vi "Load Microphone 2D Locations.vi"(3 "error in":errorcluster, 4 "Sensor Locations File":path=path "C:/Users/plane/Desktop/MTA/SCM with Cu Windows.cfg") -> (0 "error out":errorcluster, 1 "data":cluster{"r":dbl, "theta":dbl}[](array[cluster]))   [LabVIEW 2013]
panel:
  in  "Transducer Coordinates (cm, rad)":cluster{"r":dbl, "theta":dbl}[](array[cluster])
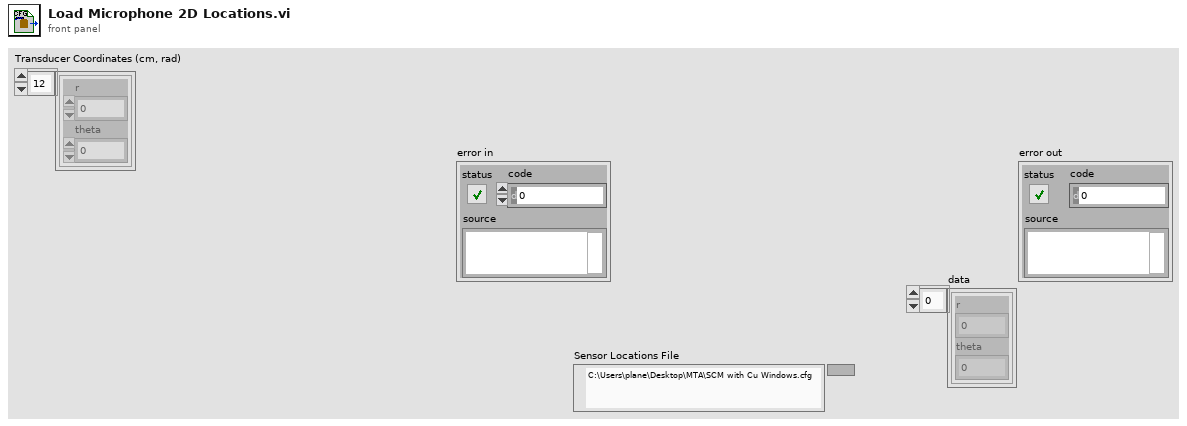
[diagram p1: front panel]
types:
  T1 = enum16{"big-endian, network order", "native, host order", "little-endian"}
  T2 = enum16{"open", "replace", "create", "open or create", "replace or create", "replace or create with confirmation"}
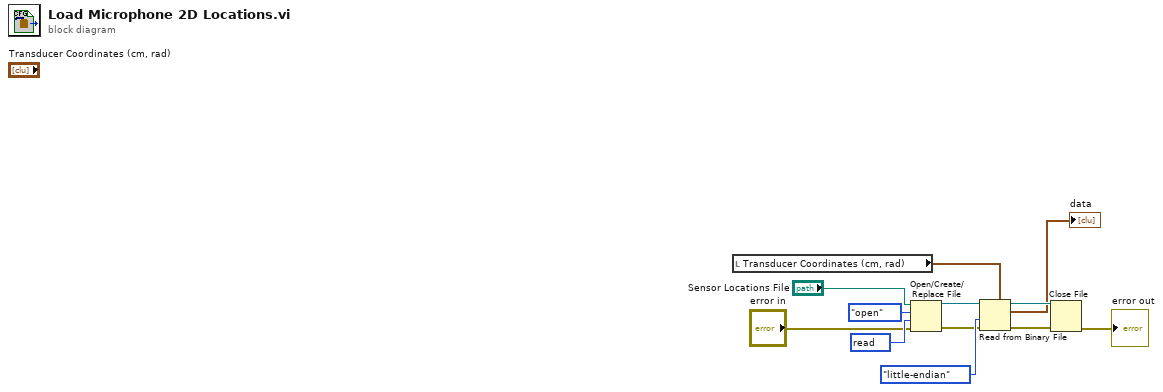
[diagram p0: block diagram]
diagram:
  w12 = u32 2147483648 items=["read"=2147483648, "write"=1073741824, "read & write"=3221225472, "execute"=536870912, "all"=268435456] ("desired access (read & write)")
  n1 = local read "Transducer Coordinates (cm, rad)"() -> (w4:cluster{"r":dbl, "theta":dbl}[])
  n2 = Open/Create/Replace File(file path (use dialog)="Sensor Locations File", error in="error in", operation (0:open)=T2."open", access (0:read/write)=w12) -> (refnum out=w8:refnum<file>, error out=w7:errorcluster)  [unwired: 2 in, 1 out]
  n3 = Read from Binary File(5:w4, 8:w7, 9:T1."little-endian" ("byte order (0:big-endian, network order)"), 11:w8) -> (0:w5:errorcluster, 2:→"data":cluster{"r":dbl, "theta":dbl}[], 3:w6:refnum<file>)  [unwired: 2 in, 1 out]
  n4 = Close File(refnum=w6, error in=w5) -> (error out=→"error out":errorcluster)  [unwired: 1 out]
